vi "Voltage - Continuous Input.vi"() -> ()   [LabVIEW 2019]
uses:
  <vilib>/DAQmx/read.llb/DAQmx Read (Analog 1D Wfm NChan NSamp).vi
  <extravilib>/ChannelInstances/Tag-bool/Read With Abort.vi
  <extravilib>/ChannelInstances/Tag-bool/Write With Abort.vi
  <vilib>/DAQmx/create/channels.llb/DAQmx Create Channel (AI-Voltage-Basic).vi
  <vilib>/DAQmx/configure/timing.llb/DAQmx Timing (Sample Clock).vi
  <extravilib>/ChannelInstances/Tag-bool/Instantiate.vi
  <extravilib>/ChannelInstances/Tag-bool/EndpointRead.vi
  <vilib>/DAQmx/miscellaneous.llb/DAQmx Fill In Error Info.vi
  <extravilib>/ChannelInstances/Tag-bool/Endpoint.vi
  <resource>/objmgr/daqmx.rc
  <extravilib>/ChannelInstances/Tag-bool.lvlib
  YAML Config Reader.lvlib
panel:
  in  "YAML configuration path":path
  out "Waveform Graph":waveform(dbl)[](graph)
  out "Waveform Graph 2":waveform(dbl)[](graph)
  out "Actual Sample Rates":dbl[](array[numeric]) format="%0.2f"
  out "error out":errorcluster
  in  "Stop":bool
  out "Waveform Graph 1":waveform(dbl)[](graph)
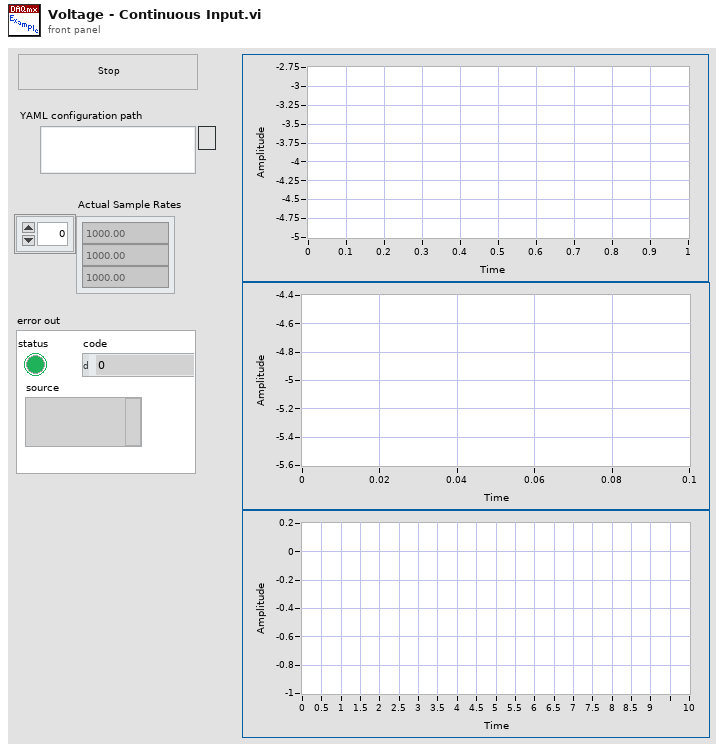
[diagram p1: front panel]
types:
  T1 = typedef "Tag-bool.lvlib/))Channel.ctl" = refnum<queue>
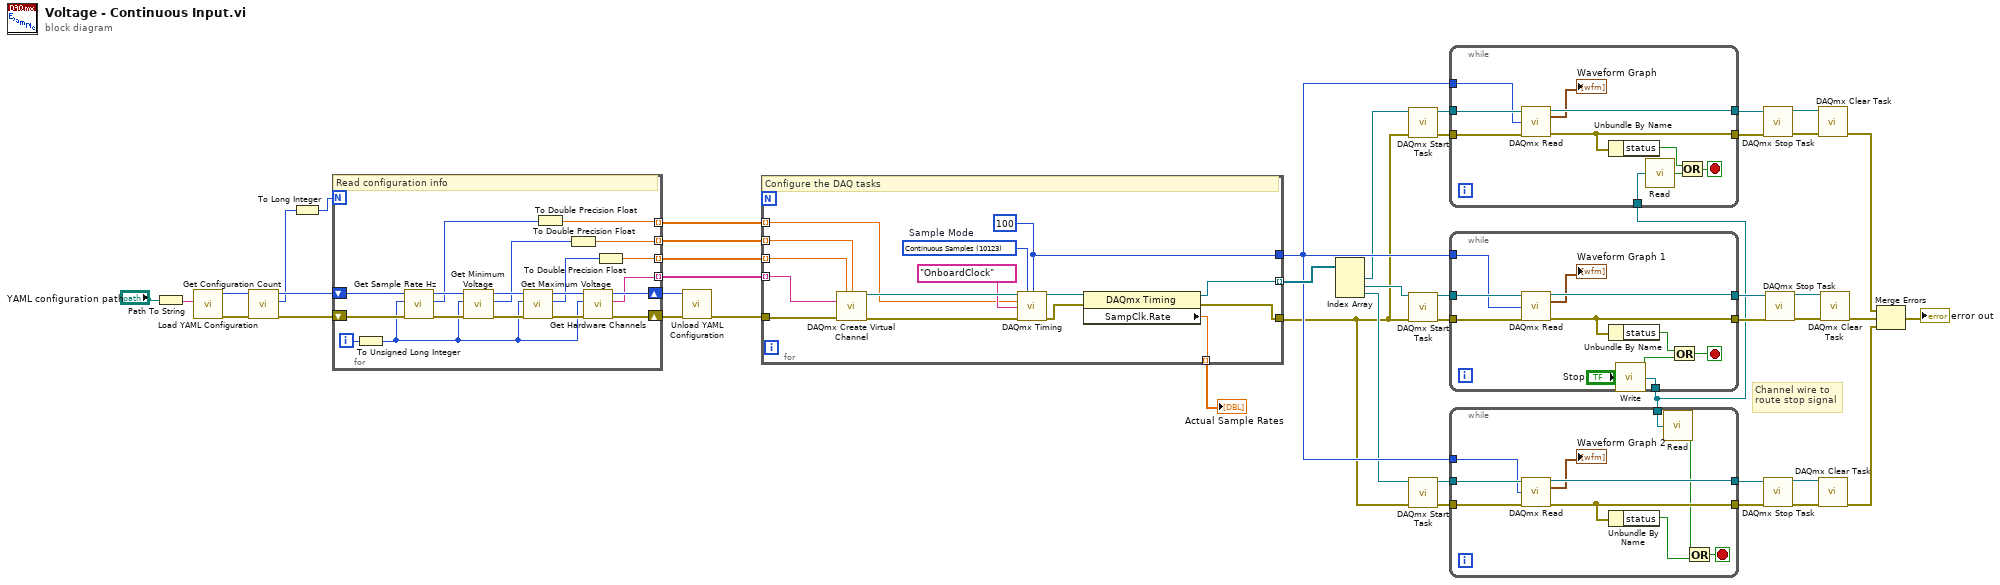
[diagram p0: block diagram]
diagram:
  # "Channel wire to route stop signal"
  n1 = Path To String(path="YAML configuration path") -> (string=w1:string)
  n2 = call "Load YAML Configuration.vi"("YAML Config File Path"=w1) -> ("Error Out"=w15:errorcluster, "YAML Handle Out"=w13:u64)  [unwired: 9 in]
  n3 = call "Get Configuration Count.vi"("Error In"=w15, "YAML Handle In"=w13) -> ("Error Out"=w14:errorcluster, "Count"=w9:i64, "YAML Handle Out"=w10:u64)  [unwired: 7 in]
  n4 = To Long Integer(number=w9) -> (32bit integer=w8:i32)
  n5 = for {
    N: w8 -> [_]
    shift-right: [w59] -> w12
    shift-left: w14 -> [w64]
    shift-right: [w58] -> w11
    shift-left: w10 -> [w56]
    tunnel: [w52] -> w7 mode=indexing
    tunnel: [w51] -> w6 mode=indexing
    tunnel: [w49] -> w5 mode=indexing
    tunnel: [w48] -> w4 mode=indexing
    i -> [w47]
    # "Read configuration info"
    n6 = To Unsigned Long Integer(number=w47) -> (unsigned 32bit integer=w46:u32)
    n7 = call "Get Sample Rate Hz.vi"("Error In"=w64, "Index"=w46, "YAML Handle In"=w56) -> ("Error Out"=w57:errorcluster, "Sample Rate (Hz)"=w54:i64, "YAML Handle Out"=w55:u64)  [unwired: 6 in]
    n8 = call "Get Minimum Voltage.vi"("Error In"=w57, "Index"=w46, "YAML Handle In"=w55) -> ("Error Out"=w63:errorcluster, "Minimum Voltage"=w53:i64, "YAML Handle Out"=w61:u64)  [unwired: 6 in]
    n9 = call "Get Maximum Voltage.vi"("Error In"=w63, "Index"=w46, "YAML Handle In"=w61) -> ("Error Out"=w62:errorcluster, "Maximum Voltage"=w50:i64, "YAML Handle Out"=w60:u64)  [unwired: 6 in]
    n10 = To Double Precision Float(number=w54) -> (double precision float=w52:dbl)
    n11 = To Double Precision Float(number=w53) -> (double precision float=w51:dbl)
    n12 = call "Get Hardware Channels.vi"("Error In"=w62, "Index"=w46, "YAML Handle In"=w60) -> ("Error Out"=w59:errorcluster, "Hardware Channels"=w48:string, "YAML Handle Out"=w58:u64)  [unwired: 6 in]
    n13 = To Double Precision Float(number=w50) -> (double precision float=w49:dbl)
  }
  n14 = call "Unload YAML Configuration.vi"("Error In"=w12, "YAML Handle In"=w11) -> ("Error Out"=w3:errorcluster)  [unwired: 9 in]
  n15 = for {
    tunnel: [w74] -> w45 mode=indexing
    tunnel: [w73] -> w16
    tunnel: w7 -> [w71] mode=indexing
    tunnel: [w70] -> w30
    tunnel: [w69] -> w39 mode=indexing
    tunnel: w4 -> [w68] mode=indexing
    tunnel: w5 -> [w67] mode=indexing
    tunnel: w6 -> [w66] mode=indexing
    tunnel: w3 -> [w65]
    w70 = 100 ("Number of Samples")
    w77 = 10123 items=["Finite Samples"=10178, "Continuous Samples"=10123, "Hardware Timed Single Point"=12522]  # Sample Mode
    # "Configure the DAQ tasks"
    n16 = call-poly <vilib>:"DAQmx Create Virtual Channel.vi"("maximum value"=w67, "minimum value"=w66, "physical channels"=w68, "error in"=w65) -> ("task out"=w75:refnum<k21>, "error out"=w76:errorcluster)  [unwired: 10 in]
    n17 = call-poly <vilib>:"DAQmx Timing.vi"("task/channels in"=w75, "sample mode"=w77, "samples per channel"=w70, "rate"=w71, "source"=tag "OnboardClock" ("Sample Clock Source"), "error in"=w76) -> ("task out"=w79:refnum<k21>, "error out"=w78:errorcluster)  [unwired: 8 in]
    n18 = property class="DAQmx Timing"(reference=w79, error in=w78) -> (reference out=w74:refnum<k21>, error out=w73:errorcluster, "SampClk.Rate"=w69:dbl)
  }
  "Actual Sample Rates" <- w39
  n19 = Index Array(array=w45) -> (element #1=w17:refnum<k21>, element #2=w20:refnum<k21>, element #3=w23:refnum<k21>)  [unwired: 3 in]
  n20 = call <vilib>:"DAQmx Start Task.vi"("task/channels in"=w17, "error in"=w16) -> ("task out"=w18:refnum<k21>, "error out"=w19:errorcluster)  [unwired: 12 in]
  n21 = call <vilib>:"DAQmx Start Task.vi"("task/channels in"=w20, "error in"=w16) -> ("task out"=w21:refnum<k21>, "error out"=w22:errorcluster)  [unwired: 12 in]
  n22 = call <vilib>:"DAQmx Start Task.vi"("task/channels in"=w23, "error in"=w16) -> ("task out"=w25:refnum<k21>, "error out"=w24:errorcluster)  [unwired: 12 in]
  n23 = while {
    tunnel: w21 -> [w89]
    tunnel: w22 -> [w88]
    tunnel: [w87] -> w43
    tunnel: [w84] -> w42
    tunnel: w30 -> [w81]
    tunnel: [w80] -> w26
    stop <- w82 stop-if-true
    n24 = call-poly <vilib>:"DAQmx Read.vi"("task/channels in"=w89, "number of samples per channel"=w81, "error in"=w88) -> ("task out"=w87:refnum<k21>, "data"=→"Waveform Graph 1":waveform(dbl)[], "error out"=w84:errorcluster)  [unwired: 10 in]
    n25 = Unbundle By Name(w84) -> ("status"=w83:bool)
    n26 = call <extravilib>:"Write.vi"("element"="Stop") -> ("channel"=w80:T1)  [unwired: 1 out]
    n27 = Or(x=w83, y="Stop") -> (x .or. y?=w82:bool)
  }
  n28 = while {
    tunnel: w18 -> [w99]
    tunnel: w19 -> [w98]
    tunnel: [w97] -> w31
    tunnel: [w95] -> w32
    tunnel: w30 -> [w92]
    tunnel: w26 -> [w90]
    stop <- w93 stop-if-true
    n29 = call-poly <vilib>:"DAQmx Read.vi"("task/channels in"=w99, "number of samples per channel"=w92, "error in"=w98) -> ("task out"=w97:refnum<k21>, "data"=→"Waveform Graph":waveform(dbl)[], "error out"=w95:errorcluster)  [unwired: 10 in]
    n30 = Unbundle By Name(w95) -> ("status"=w94:bool)
    n31 = call <extravilib>:"Read.vi"("channel"=w90) -> ("element"=w91:bool)  [unwired: 1 in, 1 out]
    n32 = Or(x=w94, y=w91) -> (x .or. y?=w93:bool)
  }
  n33 = while {
    tunnel: w25 -> [w109]
    tunnel: w24 -> [w108]
    tunnel: [w107] -> w35
    tunnel: [w105] -> w36
    tunnel: w30 -> [w102]
    tunnel: w26 -> [w100]
    stop <- w103 stop-if-true
    n34 = call-poly <vilib>:"DAQmx Read.vi"("task/channels in"=w109, "number of samples per channel"=w102, "error in"=w108) -> ("task out"=w107:refnum<k21>, "data"=→"Waveform Graph 2":waveform(dbl)[], "error out"=w105:errorcluster)  [unwired: 10 in]
    n35 = Unbundle By Name(w105) -> ("status"=w104:bool)
    n36 = call <extravilib>:"Read.vi"("channel"=w100) -> ("element"=w101:bool)  [unwired: 1 in, 1 out]
    n37 = Or(x=w101, y=w104) -> (x .or. y?=w103:bool)
  }
  n38 = call <vilib>:"DAQmx Stop Task.vi"("task/channels in"=w31, "error in"=w32) -> ("task out"=w34:refnum<k21>, "error out"=w33:errorcluster)  [unwired: 12 in]
  n39 = call <vilib>:"DAQmx Stop Task.vi"("task/channels in"=w35, "error in"=w36) -> ("task out"=w38:refnum<k21>, "error out"=w37:errorcluster)  [unwired: 12 in]
  n40 = call <vilib>:"DAQmx Stop Task.vi"("task/channels in"=w43, "error in"=w42) -> ("task out"=w40:refnum<k21>, "error out"=w41:errorcluster)  [unwired: 12 in]
  n41 = call <vilib>:"DAQmx Clear Task.vi"("task in"=w34, "error in"=w33) -> ("error out"=w28:errorcluster)  [unwired: 13 in]
  n42 = call <vilib>:"DAQmx Clear Task.vi"("task in"=w38, "error in"=w37) -> ("error out"=w27:errorcluster)  [unwired: 13 in]
  n43 = call <vilib>:"DAQmx Clear Task.vi"("task in"=w40, "error in"=w41) -> ("error out"=w44:errorcluster)  [unwired: 13 in]
  n44 = Merge Errors(w28, w44, w27) -> (→"error out":errorcluster)
